vi "sys_get.vi"(8 "error in":errorcluster, 9 "address":string, 10 "Sys get command":u16(ring) items=["version", "nvm", "vdd", "hweui"], 11 "VISA in":refnum<visa-resource-name>) -> (0 "error out":errorcluster, 2 "response":string="\r\n", 3 "VISA out":refnum<visa-resource-name>)   [LabVIEW 2011]
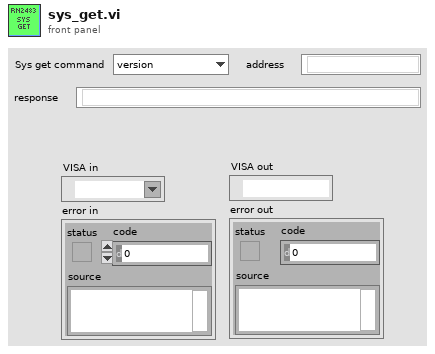
[diagram p1: front panel]
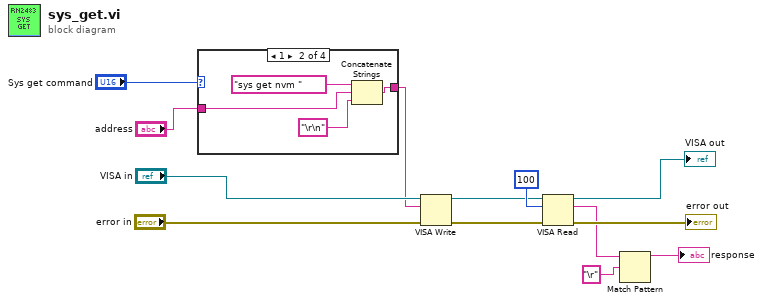
[diagram p0: block diagram]
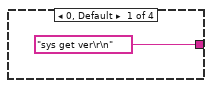
[diagram p2: hidden frame]
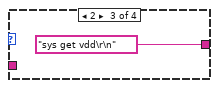
[diagram p3: hidden frame]
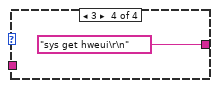
[diagram p4: hidden frame]
diagram:
  n1 = case shown="1" "Sys get command" {
    tunnel: ["sys get ver\r\n" ("string to write") w18 "sys get vdd\r\n" ("string to write") "sys get hweui\r\n" ("string to write")] -> w6
    tunnel: "address" -> [_ w15 _ _]
    frame 0, Default {
    }
    frame 1 {
      n2 = Concatenate Strings("sys get nvm " ("string to write"), w15, "\r\n" ("string to write")) -> (w18:string)
    }
    frame 2 {
    }
    frame 3 {
    }
  }
  n3 = VISA Write(VISA resource name="VISA in", write buffer=w6, error in (no error)="error in") -> (VISA resource name out=w8:refnum<visa-resource-name>, error out=w7:errorcluster)  [unwired: 1 out]
  n4 = VISA Read(VISA resource name=w8, byte count=u32 100, error in (no error)=w7) -> (VISA resource name out=→"VISA out":refnum<visa-resource-name>, read buffer=w2:string, error out=→"error out":errorcluster)  [unwired: 1 out]
  n5 = Match Pattern(string=w2, regular expression="\r" ("string to write")) -> (before substring=→"response":string)  [unwired: 1 in, 3 out]
